vi "Test NI Camera.vi"() -> ()   [LabVIEW 2014]
uses:
  NI Camera Functions.ctl
panel:
  in  "Stop Acquisition":bool
  in  "Start Acquisition":bool
  in  "Stop":bool
  out "Frame Rate":dbl
  out "Image":T1(plugin-control)
  out "Buffer Number":u32
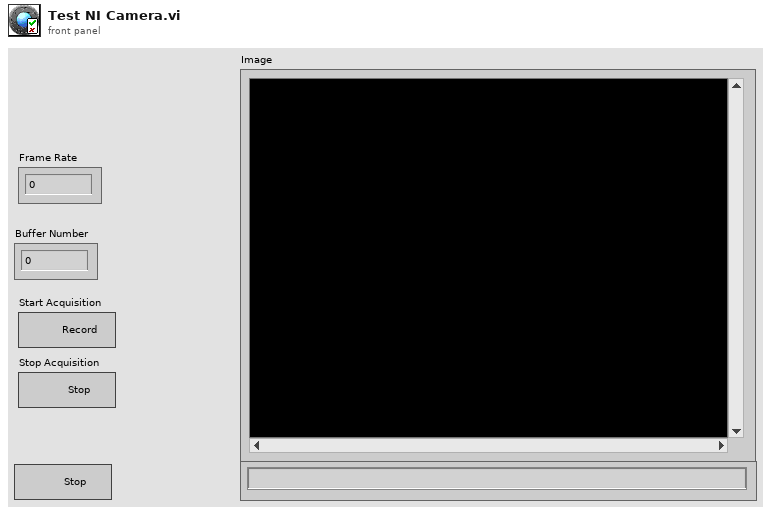
[diagram p1: front panel]
types:
  T1 = typedef "IMAQ Image.ctl" = refnum<image>
  T2 = typedef "NI Camera Functions.ctl" = enum16{"Connect", "Disconnect", "Start Live", "Stop Live", "Acquire", "Update Refnums"}
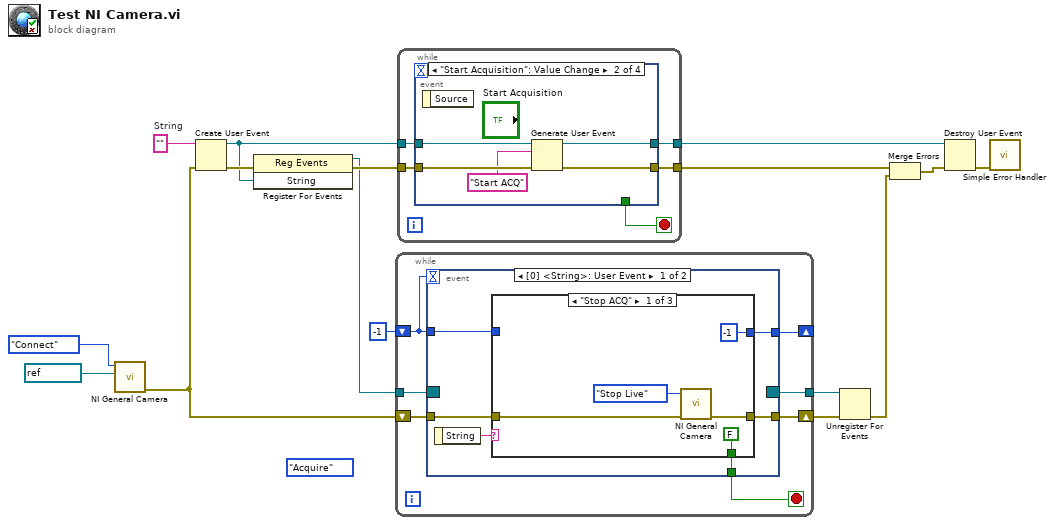
[diagram p0: block diagram]
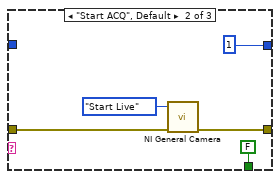
[diagram p2: hidden frame]
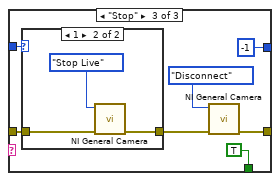
[diagram p3: hidden frame]
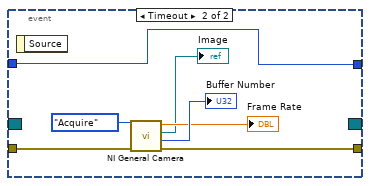
[diagram p5: hidden frame]
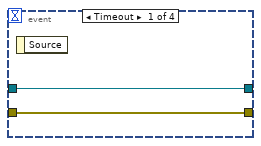
[diagram p6: hidden frame]
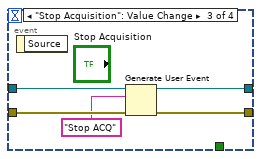
[diagram p7: hidden frame]
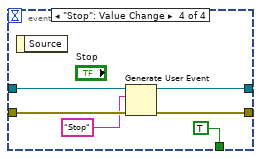
[diagram p8: hidden frame]
diagram:
  (unwired) NI_Camera_Functions."Acquire" ("Function")
  w3 = ""  # String
  n1 = call "NI General Camera.vi"("Camera Name"=refnum<k21> "cam0", "Function"=NI_Camera_Functions."Connect") -> ("error out"=w11:errorcluster)  [unwired: 6 in, 3 out]
  n2 = Create User Event(user event datatype=w3, error in=w11) -> (user event=w15:refnum<user-event>, error out=w16:errorcluster)
  n3 = register-events(error in=w16, w15) -> (reference out=w13:refnum<event-registration>, error out=w14:errorcluster)  [unwired: 1 in]
  n4 = while {
    shift-right: [w21] -> w9
    shift-left: w11 -> [w22]
    tunnel: w13 -> [w23]
    tunnel: [w20] -> w8
    shift-right: [w18] -> _
    shift-left: -1 -> [w17]
    stop <- w19 stop-if-true
    n5 = event shown="[0] <String>: User Event" {
      selector: w23 -> [_ _]
      dyn-events: [_ _] -> w20
      timeout: w17 -> [_ _]
      tunnel: w22 -> [w28 w53]
      tunnel: [w29 w54] -> w21
      tunnel: [w27 _] -> w19
      tunnel: [w25 w52] -> w18
      tunnel: w17 -> [w24 w52]
      event User Event {
        n6 = event-data() -> ("String"=w26:string)  [unwired: 1 in]
        n7 = case shown="\"Stop ACQ\"" w26 {
          tunnel: w28 -> [w32 w37 w41]
          tunnel: [w33 w36 w45] -> w29
          tunnel: [FALSE FALSE TRUE] -> w27
          tunnel: [-1 1 -1] -> w25
          tunnel: w24 -> [_ _ w42]
          frame "Stop ACQ" {
            n8 = call "NI General Camera.vi"("error in (no error)"=w32, "Function"=NI_Camera_Functions."Stop Live") -> ("error out"=w33:errorcluster)  [unwired: 6 in, 3 out]
          }
          frame "Start ACQ", Default {
            n9 = call "NI General Camera.vi"("error in (no error)"=w37, "Function"=NI_Camera_Functions."Start Live") -> ("error out"=w36:errorcluster)  [unwired: 6 in, 3 out]
          }
          frame "Stop" {
            n10 = case shown="1" w42 {
              tunnel: w41 -> [w47 w49]
              tunnel: [w47 w48] -> w40
              frame 0, Default {
              }
              frame 1 {
                n11 = call "NI General Camera.vi"("error in (no error)"=w49, "Function"=NI_Camera_Functions."Stop Live") -> ("error out"=w48:errorcluster)  [unwired: 6 in, 3 out]
              }
            }
            n12 = call "NI General Camera.vi"("error in (no error)"=w40, "Function"=NI_Camera_Functions."Disconnect") -> ("error out"=w45:errorcluster)  [unwired: 6 in, 3 out]
          }
        }
      }
      event Timeout {
        n13 = event-data() -> ()  [unwired: 1 in, 1 out]
        n14 = call "NI General Camera.vi"("error in (no error)"=w53, "Function"=NI_Camera_Functions."Acquire") -> ("error out"=w54:errorcluster, "Buffer Number"=→"Buffer Number":u32, "Image"=→"Image":T1, "Frame Rate"=→"Frame Rate":dbl)  [unwired: 6 in]
      }
    }
  }
  n15 = while {
    tunnel: w14 -> [w61]
    tunnel: w15 -> [w60]
    tunnel: [w62] -> w6
    tunnel: [w59] -> w10
    stop <- w58 stop-if-true
    n16 = event shown="[1] \"Start Acquisition\": Value Change" {
      selector: _ -> [_ _ _ _]
      dyn-events: _ -> [_ _ _ _]
      timeout: _ -> [_ _ _ _]
      tunnel: [w63 w68 w73 w79] -> w62
      tunnel: w61 -> [w63 w69 w74 w80]
      tunnel: w60 -> [w64 w67 w72 w78]
      tunnel: [w64 w66 w71 w77] -> w59
      tunnel: [_ _ _ TRUE] -> w58
      event Timeout {
        n17 = event-data() -> ()  [unwired: 1 in, 1 out]
      }
      event "Start Acquisition": Value Change {
        n18 = event-data() -> ()  [unwired: 1 in, 1 out]
        n19 = Generate User Event(user event=w67, event data cluster="Start ACQ", error in=w69) -> (user event out=w66:refnum<user-event>, error out=w68:errorcluster)  [unwired: 1 in]
      }
      event "Stop Acquisition": Value Change {
        n20 = event-data() -> ()  [unwired: 1 in, 1 out]
        n21 = Generate User Event(user event=w72, event data cluster="Stop ACQ", error in=w74) -> (user event out=w71:refnum<user-event>, error out=w73:errorcluster)  [unwired: 1 in]
      }
      event "Stop": Value Change {
        n22 = event-data() -> ()  [unwired: 1 in, 1 out]
        n23 = Generate User Event(user event=w78, event data cluster="Stop", error in=w80) -> (user event out=w77:refnum<user-event>, error out=w79:errorcluster)  [unwired: 1 in]
      }
    }
  }
  n24 = Unregister For Events(event registration refnum=w8, error in=w9) -> (error out=w7:errorcluster)
  n25 = Merge Errors(w6, w7) -> (w4:errorcluster)
  n26 = Destroy User Event(user event=w10, error in=w4) -> (error out=w5:errorcluster)
  n27 = call <vilib>:"Simple Error Handler.vi"("error in (no error)"=w5) -> ()  [unwired: 4 in, 5 out]
